vi "Search all lines of CSV file string for value.vi"(0 "Compare value":string, 5 "CSV file string":string, 7 "CSV field (0-n)":i32, 11 "error in":errorcluster) -> (4 "Found value":bool, 15 "error out":errorcluster)   [LabVIEW 2013]
doc: "This vi will search all lines of a csv file for a certain value in a certain field (0 based)"
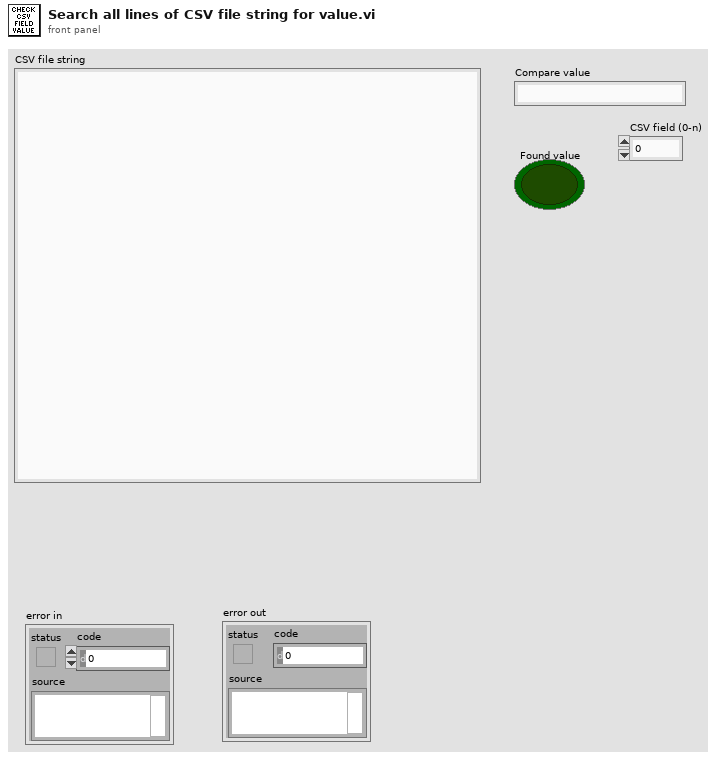
[diagram p1: front panel]
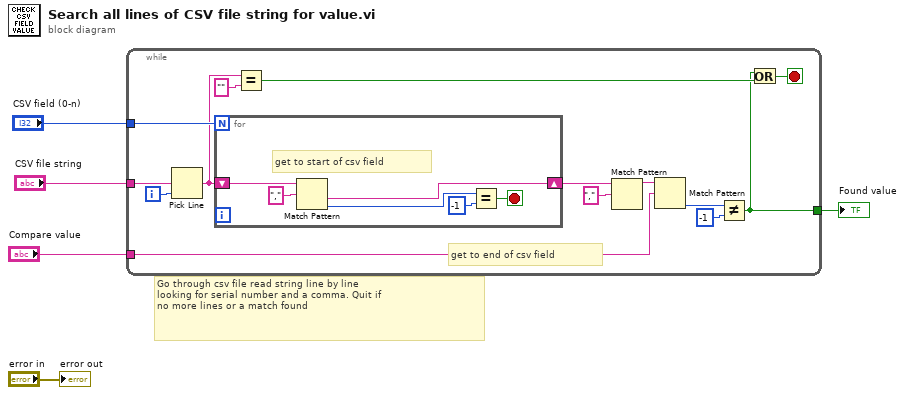
[diagram p0: block diagram]
diagram:
  # "Go through csv file read string line by line\nlooking for serial number and a comma. Quit if\nno more lines or a match found"
  n1 = while {
    tunnel: "CSV file string" -> [w19]
    tunnel: "Compare value" -> [w16]
    tunnel: [w11] -> w2
    tunnel: "CSV field (0-n)" -> [w10]
    i -> [w18]
    stop <- w12 stop-if-true
    # "get to end of csv field"
    n2 = Pick Line(multi-line string=w19, line index=w18) -> (output string=w9:string)  [unwired: 1 in]
    n3 = for {
      N: w10 -> [_]
      shift-right: [w20] -> w7
      shift-left: w9 -> [w25]
      stop <- w21 stop-if-true
      # "get to start of csv field"
      n4 = Match Pattern(string=w25, regular expression=",") -> (after substring=w20:string, offset past match=w22:i32)  [unwired: 1 in, 2 out]
      n5 = Equal?(x=w22, y=-1) -> (x = y?=w21:bool)
    }
    n6 = Equal?(x=w9, y="") -> (x = y?=w13:bool)
    n7 = Match Pattern(string=w7, regular expression=",") -> (before substring=w6:string)  [unwired: 1 in, 3 out]
    n8 = Match Pattern(string=w6, regular expression=w16) -> (offset past match=w15:i32)  [unwired: 1 in, 3 out]
    n9 = Not Equal?(x=w15, y=-1) -> (x != y?=w11:bool)
    n10 = Or(x=w11, y=w13) -> (x .or. y?=w12:bool)
  }
  "Found value" <- w2
  "error out" <- "error in"
